vi "rad_Configure Discovery Settings Dialog.vi"(11 "Discovery Settings":T2 {"Targets Information"."Primary NIC"."IP Address Request Mode" items=["Static"=1, "DHCP/Link-Local"=2, "Link-Local Only"=4, "DHCP Only"=8]}) -> (1 "Changes?":bool, 3 "Discovery Settings out":T2 {"Targets Information"."Primary NIC"."IP Address Request Mode" items=["Static"=1, "DHCP/Link-Local"=2, "Link-Local Only"=4, "DHCP Only"=8]})   [LabVIEW 2020]
doc: "Dialog that allows the user to configure the method that will be used to add targets from the network."
uses:
  TypeDefs/rad_State Data.ctl
  TypeDefs/rad_Targets Settings.ctl
  support/New folder/Target Information.ctl
  TypeDefs/rad_Target Network Settings.ctl
  support/Controls/Discovery Settings.ctl
  support/Controls/Discovery Method Enum.ctl
  support/Controls/Important Paths.ctl
  Util/FP Control/FP Control Functions.ctl
panel:
  in  "Discovery.Method":T1=enum."IPsFile"
  in  "PathFile":path
  in  "NotAsk":bool
  in  "Cancel":bool
  in  "OK":bool
  # "Choose the method to add targets from the Network"
  # "*This will also affect the Refresh Button Behavior"
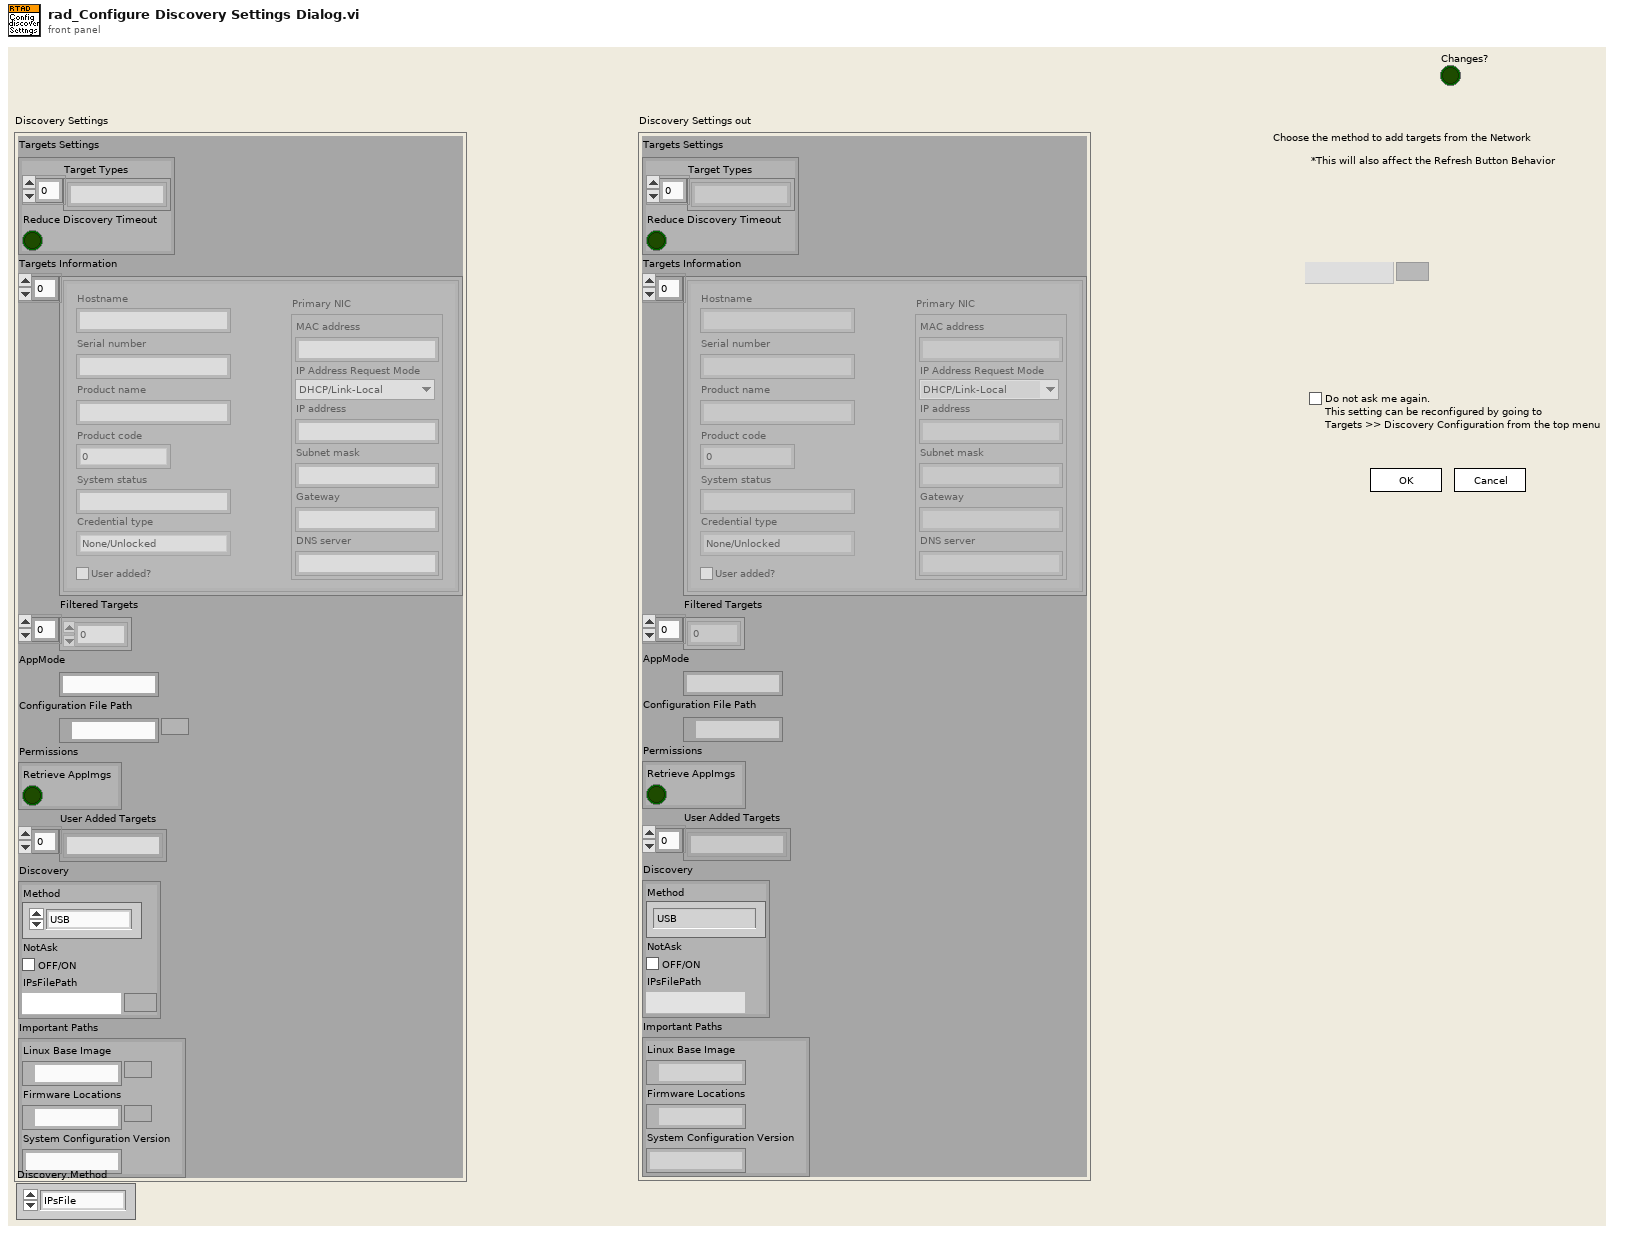
[diagram p1: front panel]
types:
  T1 = typedef "Discovery Method Enum.ctl" = enum32{"USB", "IPsFile", "AutoAll", "NotDiscover"}
  T2 = typedef "rad_State Data.ctl" = cluster{"Targets Settings":T3, "Targets Information":T4[], "Filtered Targets":i32[], "AppMode":string, "Configuration File Path":path, "Permissions":cluster{"Retrieve AppImgs":bool}, "User Added Targets":string[], "Discovery":T6, "Important Paths":T7}
  T3 = typedef "rad_Targets Settings.ctl" = cluster{"Target Types":string[], "Reduce Discovery Timeout":bool}
  T4 = typedef "Target Information.ctl" = cluster{"Hostname":string, "Serial number":string, "Product name":string, "Product code":i32, "System status":string, "Credential type":enum16{"None/Unlocked", "FTP Password", "NIAuth Credentials"}, "User added?":bool, "Primary NIC":T5}
  T5 = typedef "rad_Target Network Settings.ctl" = cluster{"MAC address":string, "IP Address Request Mode":i32, "IP address":string, "Subnet mask":string, "Gateway":string, "DNS server":string}
  T6 = typedef "Discovery Settings.ctl" = cluster{"Method":T1, "NotAsk":bool, "IPsFilePath":path}
  T7 = typedef "Important Paths.ctl" = cluster{"Linux Base Image":path, "Firmware Locations":path, "System Configuration Version":string}
  T8 = typedef "FP Control Functions.ctl" = enum16{"Open", "Close", "Bring To Front", "Center"}
  T9 = enum8{"Enabled", "Disabled", "Disabled and Grayed Out"}
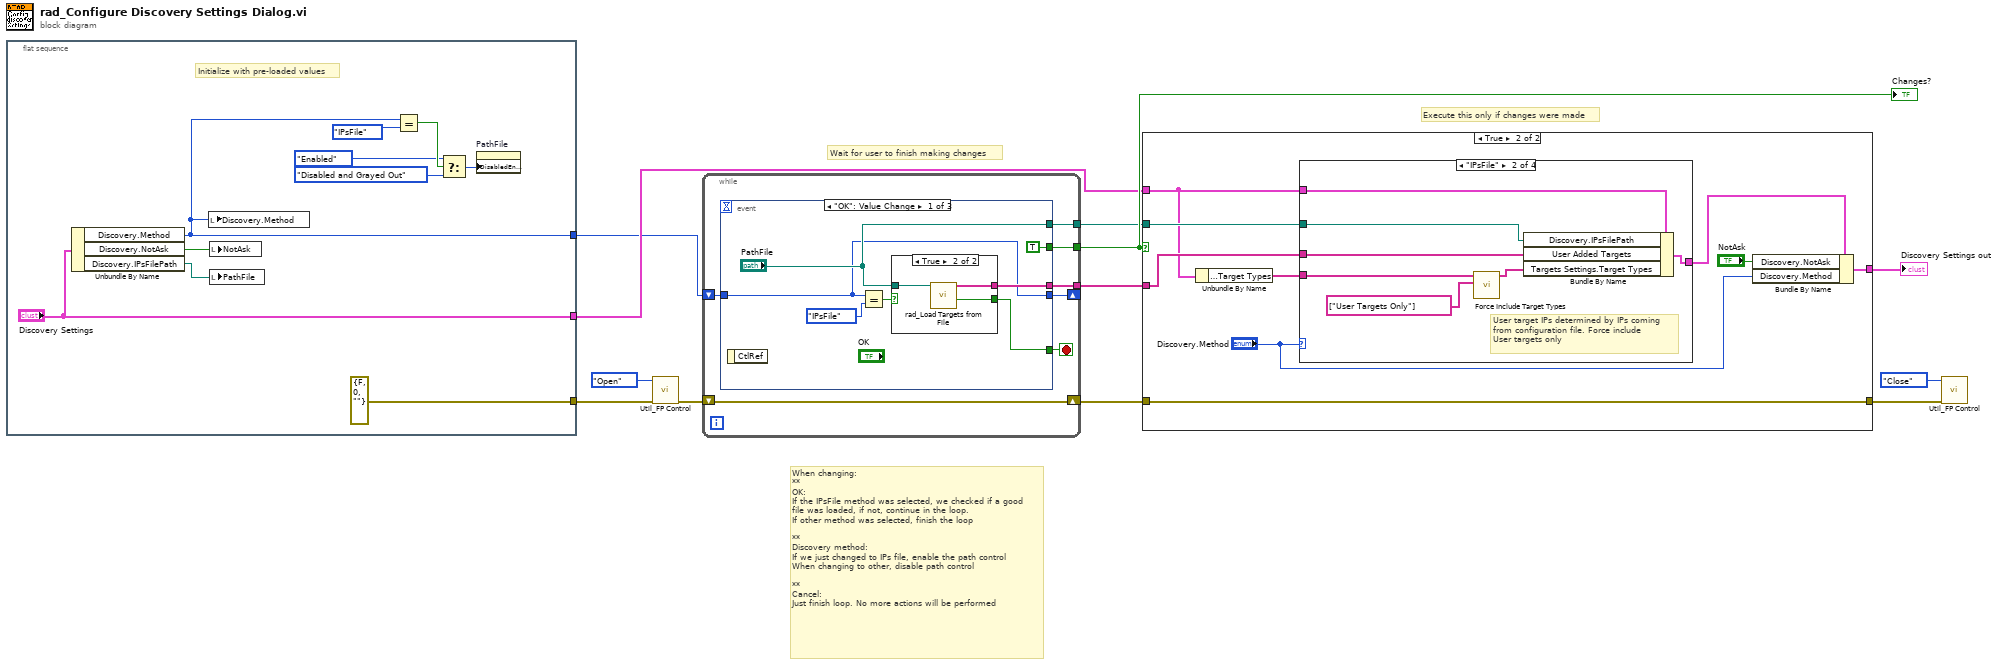
[diagram p0: block diagram]
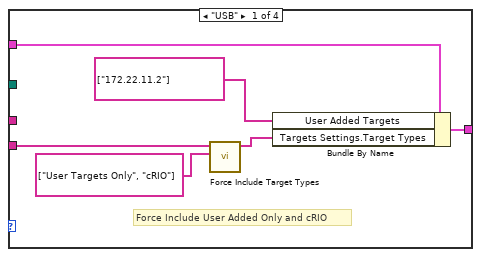
[diagram p3: hidden frame]
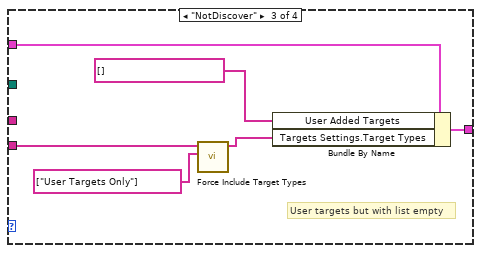
[diagram p4: hidden frame]
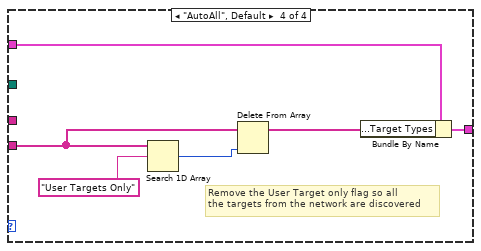
[diagram p5: hidden frame]
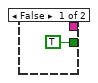
[diagram p6: hidden frame]
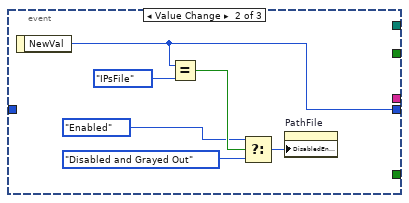
[diagram p7: hidden frame]
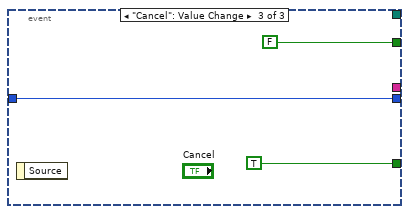
[diagram p8: hidden frame]
diagram:
  # "When changing:\n**\nOK:\nIf the IPsFile method was selected, we checked if a good\nfile was loaded, if not, continue in the loop.\nIf other method was selected, finish the loop\n\n**\nDiscovery method:\nIf we just changed to IPs file, enable the path control\nWhen changing to other, disable path control\n\n**\nCancel:\nJust finish loop. No more actions will be performed"
  # "Wait for user to finish making changes"
  # "Execute this only if changes were made"
  n1 = flat-sequence {
    tunnel: [errorcluster {"status"=FALSE, "code"=0, "source"=""} ("error constant")] -> w11
    tunnel: ["Discovery Settings"] -> w4
    tunnel: [w13] -> w1
    frame #0 {
      # "Initialize with pre-loaded values"
      n2 = Unbundle By Name("Discovery Settings") -> ("Discovery.Method"=w13:T1, "Discovery.NotAsk"=w22:bool, "Discovery.IPsFilePath"=w15:path)
      n3 = local write "Discovery.Method"(w13) -> ()
      n4 = local write "NotAsk"(w22) -> ()
      n5 = local write "PathFile"(w15) -> ()
      n6 = Equal?(x=w13, y=Discovery_Method_Enum."IPsFile" ("Discovery.Method")) -> (x = y?=w19:bool)
      n7 = Select(t=T9."Enabled", s=w19, f=T9."Disabled and Grayed Out" ("Disabled")) -> (s? t:f=w18:T9)
      n8 = property on="PathFile" class="Path"("DisabledEnum"=w18) -> ()  [unwired: 2 in, 2 out]
    }
  }
  n9 = call "Util_FP Control.vi"("error in (no error)"=w11, "Function"=FP_Control_Functions."Open") -> ("error out"=w10:errorcluster)  [unwired: 9 out]
  n10 = while {
    shift-right: [w29] -> w7
    shift-left: w10 -> [w29]
    tunnel: [w27] -> w9
    shift-right: [w26] -> _
    shift-left: w1 -> [w25]
    tunnel: [w24] -> w3
    tunnel: [w23] -> w2
    stop <- w28 stop-if-true
    n11 = event shown="[0] \"OK\": Value Change" {
      selector: _ -> [_ _ _]
      dyn-events: _ -> [_ _ _]
      timeout: _ -> [_ _ _]
      tunnel: [w34 _ TRUE] -> w28
      tunnel: [TRUE _ FALSE] -> w27
      tunnel: [w30 w42 w47] -> w26
      tunnel: w25 -> [w30 _ w47]
      tunnel: [w33 _ _] -> w24
      tunnel: ["PathFile" _ _] -> w23
      event "OK": Value Change {
        n12 = event-data() -> ()  [unwired: 1 in, 1 out]
        n13 = Equal?(x=w30, y=Discovery_Method_Enum."IPsFile" ("Discovery.Method")) -> (x = y?=w35:bool)
        n14 = case shown="True" w35 {
          tunnel: "PathFile" -> [_ w40]
          tunnel: [TRUE ("Valid File") w39] -> w34
          tunnel: [_ w38] -> w33
          frame False {
          }
          frame True {
            n15 = call "rad_Load Targets from File.vi"("PathFile"=w40) -> ("Valid File"=w39:bool, "IPs to Load"=w38:string[])  [unwired: 9 in]
          }
        }
      }
      event Value Change {
        n16 = event-data() -> ("NewVal"=w42:T1)  [unwired: 1 in]
        n17 = Equal?(x=w42, y=Discovery_Method_Enum."IPsFile" ("Discovery.Method")) -> (x = y?=w44:bool)
        n18 = Select(t=T9."Enabled", s=w44, f=T9."Disabled and Grayed Out" ("Disabled")) -> (s? t:f=w46:T9)
        n19 = property on="PathFile" class="Path"("DisabledEnum"=w46) -> ()  [unwired: 2 in, 2 out]
      }
      event "Cancel": Value Change {
        n20 = event-data() -> ()  [unwired: 1 in, 1 out]
      }
    }
  }
  "Changes?" <- w9
  n21 = case shown="True" w9 {
    tunnel: w4 -> [w51 w54]
    tunnel: [w51 w59] -> w8
    tunnel: [w50 w57] -> w6
    tunnel: w7 -> [w50 w57]
    tunnel: w3 -> [_ w56]
    tunnel: w2 -> [_ w55]
    frame False {
    }
    frame True {
      n22 = Unbundle By Name(w54) -> ("Targets Settings.Target Types"=w53:string[])
      n23 = case shown="\"IPsFile\"" "Discovery.Method" {
        tunnel: w54 -> [w66 w73 w79 w85]
        tunnel: [w65 w72 w78 w84] -> w60
        tunnel: w56 -> [_ w71 _ _]
        tunnel: w55 -> [_ w70 _ _]
        tunnel: w53 -> [w63 w69 w75 w82]
        frame "USB" {
          # "Force Include User Added Only and cRIO"
          n24 = call "Force Include Target Types.vi"("Target Types to include"=string[] ["User Targets Only", "cRIO"] ("Targets Settings.Target Types"), "Original Target Types"=w63) -> ("Final Target Types"=w62:string[])  [unwired: 9 in]
          n25 = Bundle By Name(cluster=w66, "User Added Targets"=string[] ["172.22.11.2"], "Targets Settings.Target Types"=w62) -> (w65:T2)
        }
        frame "IPsFile" {
          # "User target IPs determined by IPs coming\nfrom configuration file. Force include\nUser targets only"
          n26 = call "Force Include Target Types.vi"("Target Types to include"=string[] ["User Targets Only"] ("Targets Settings.Target Types"), "Original Target Types"=w69) -> ("Final Target Types"=w68:string[])  [unwired: 9 in]
          n27 = Bundle By Name(cluster=w73, "Discovery.IPsFilePath"=w70, "User Added Targets"=w71, "Targets Settings.Target Types"=w68) -> (w72:T2)
        }
        frame "NotDiscover" {
          # "User targets but with list empty"
          n28 = call "Force Include Target Types.vi"("Target Types to include"=string[] ["User Targets Only"] ("Targets Settings.Target Types"), "Original Target Types"=w75) -> ("Final Target Types"=w74:string[])  [unwired: 9 in]
          n29 = Bundle By Name(cluster=w79, "User Added Targets"=string[] [], "Targets Settings.Target Types"=w74) -> (w78:T2)
        }
        frame "AutoAll", Default {
          # "Remove the User Target only flag so all\nthe targets from the network are discovered"
          n30 = Search 1D Array(1D array=w82, element="User Targets Only") -> (index of element=w81:i32)  [unwired: 1 in]
          n31 = Delete From Array "Delete From Array"(array=w82, index=w81) -> (array with subset deleted=w80:string[])  [unwired: 1 in, 1 out]
          n32 = Bundle By Name(cluster=w85, "Targets Settings.Target Types"=w80) -> (w84:T2)
        }
      }
      n33 = Bundle By Name(cluster=w60, "Discovery.NotAsk"="NotAsk", "Discovery.Method"="Discovery.Method") -> (w59:T2)
    }
  }
  "Discovery Settings out" <- w8
  n34 = call "Util_FP Control.vi"("error in (no error)"=w6, "Function"=FP_Control_Functions."Close") -> ()  [unwired: 10 out]
